vi "ZCAN_StartCAN.vi"(8 "error in (no error)":errorcluster caption="错误输入（无错误）", 10 "can_index_handle":u64) -> (0 "error out":errorcluster caption="错误输出", 1 "can_index_handle(out)":u64, 2 "startcan_success?":bool)   [LabVIEW 2018, in "zlgcan.lvlib"]
doc: "该函数用于启动CAN通道。"
uses:
  zlgcan.lvlib
  bin/ControlCANFD.dll
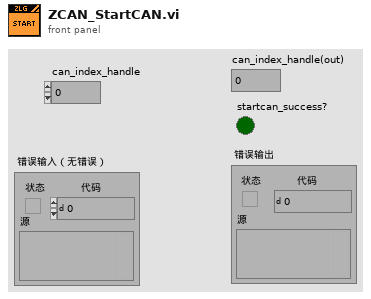
[diagram p1: front panel]
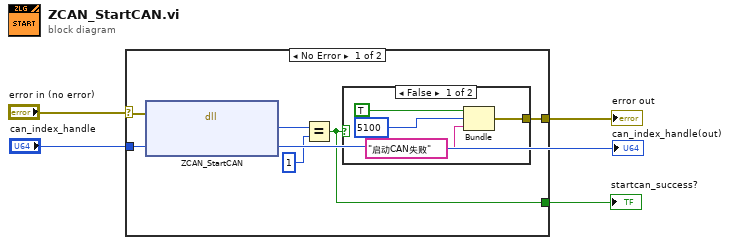
[diagram p0: block diagram]
diagram:
  n1 = case shown="No Error" "error in (no error)" {
    selector: "error in (no error)" -> [w8 w15]
    tunnel: [w6 w15] -> w3
    tunnel: "can_index_handle" -> [w7 _]
    tunnel: [w5 _] -> w2
    frame No Error {
      n2 = dll-call lib="C:/Users/ttc52/Desktop/DHC FD LV2018/LABIVIEW CANFD Tool_V1.2.4_20220724/bin/ControlCANFD.dll" fn="ZCAN_StartCAN"(error in=w8, "can_handle"=w7) -> ("return"=w10:u32)  [unwired: 3 in, 2 out]
      n3 = Equal?(x=w10, y=1) -> (x = y?=w5:bool)
      n4 = case shown="False" w5 {
        tunnel: [w11 _] -> w6
        frame False {
          n5 = Bundle("status"=TRUE, "code"=5100, "消息"="启动CAN失败") -> (w11:cluster{"status":bool, "code":i32, "消息":string})  [unwired: 1 in]
        }
        frame True {
        }
      }
    }
    frame Error {
    }
  }
  "error out" <- w3
  "startcan_success?" <- w2
  "can_index_handle(out)" <- "can_index_handle"
